vi "verify parameters in range.vi"(8 "error in (no error)":errorcluster, 11 "Simulated_CCD_Camera in":refnum<class "Simulated Camera.lvclass">) -> (0 "error out":errorcluster, 3 "Simulated_CCD_Camera out":refnum<class "Simulated Camera.lvclass">)   [LabVIEW 2018, in "Simulated Camera.lvclass"]
doc: "Verify if the parameters of the camera are in range\n\nThe operating parameters of the CCDs must be within a predefined range. This function verifies if the values provided for these parameters meet this specification. If not, ACS will not allow to start an exposure."
uses:
  Simulated Camera.lvclass
  Simulated Camera.lvclass/Simulated Camera.ctl
panel:
  out "new operation mode":T1
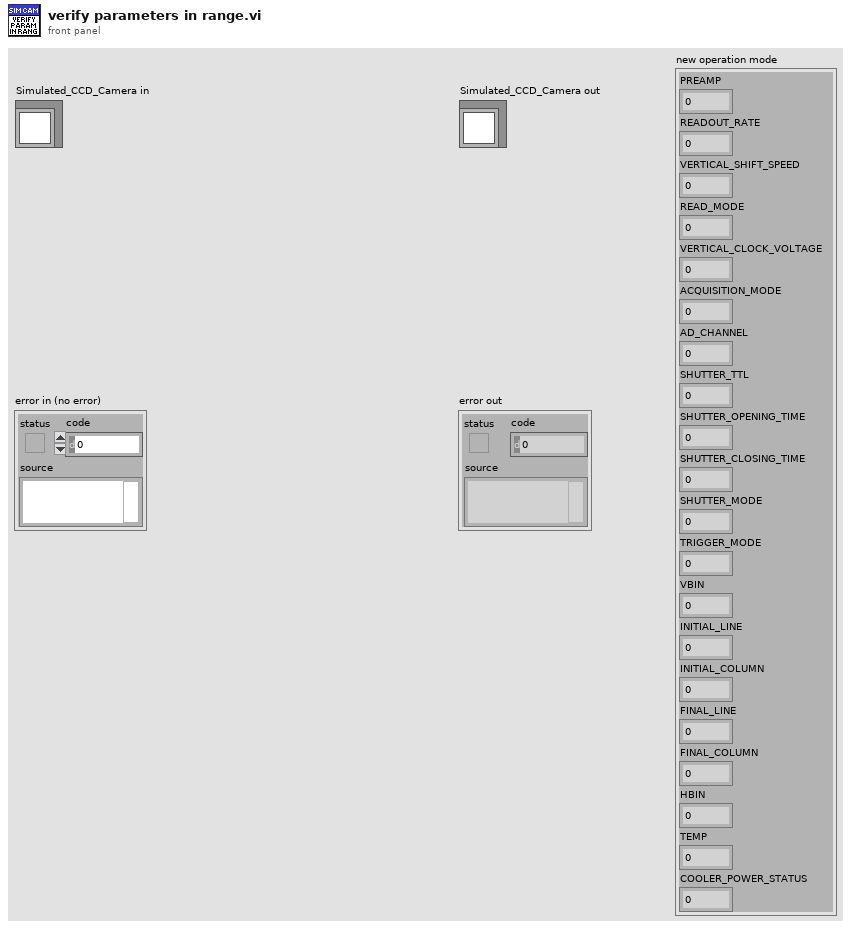
[diagram p1: front panel]
types:
  T1 = cluster{"PREAMP":u16, "READOUT_RATE":u16, "VERTICAL_SHIFT_SPEED":u16, "READ_MODE":u16, "VERTICAL_CLOCK_VOLTAGE":u16, "ACQUISITION_MODE":u16, "AD_CHANNEL":u16, "SHUTTER_TTL":u16, "SHUTTER_OPENING_TIME":u16, "SHUTTER_CLOSING_TIME":u16, "SHUTTER_MODE":u16, "TRIGGER_MODE":u16, "VBIN":u16, "INITIAL_LINE":u16, "INITIAL_COLUMN":u16, "FINAL_LINE":u16, "FINAL_COLUMN":u16, "HBIN":u16, "TEMP":u16, "COOLER_POWER_STATUS":u16}
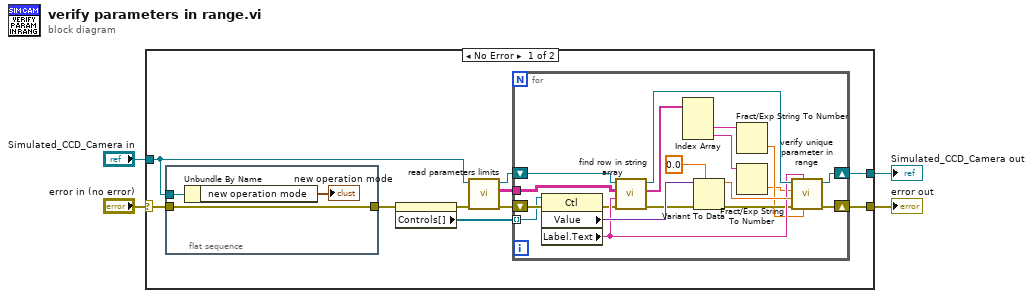
[diagram p0: block diagram]
diagram:
  n1 = case shown="No Error" "error in (no error)" {
    selector: "error in (no error)" -> [w8 w38]
    tunnel: [w14 w38] -> w3
    tunnel: [w13 w37] -> w2
    tunnel: "Simulated_CCD_Camera in" -> [w12 w37]
    frame No Error {
      n2 = flat-sequence {
        tunnel: w12 -> [w17]
        tunnel: w8 -> [w15]
        tunnel: [w15] -> w7
        frame #0 {
          n3 = Unbundle By Name(w17) -> ("new operation mode"=→"new operation mode":T1)
        }
      }
      n4 = property on="new operation mode" class="Clust (strict)"(error in=w7) -> (error out=w6:errorcluster, "Controls[]"=w5:refnum<vi>[])  [unwired: 1 in, 1 out]
      n5 = call "read parameters limits.vi"("error in (no error)"=w6, "Simulated_CCD_Camera in"=w12) -> ("error out"=w11:errorcluster, "limit values spreadsheet"=w10:string[][], "Simulated_CCD_Camera out"=w9:refnum<class "Simulated Camera.lvclass">)  [unwired: 7 in]
      n6 = for {
        shift-right: [w36] -> w14
        shift-left: w11 -> [w21]
        tunnel: w10 -> [w31]
        shift-right: [w32] -> w13
        shift-left: w9 -> [w29]
        tunnel: w5 -> [w18] mode=indexing
        n7 = property class="Ctl"(reference=w18, error in=w21) -> (error out=w23:errorcluster, "Value"=w35:variant, "Label.Text"=w25:string)  [unwired: 1 out]
        n8 = call "find row in string array.vi"("error in (no error)"=w23, "parameter name"=w25, "limit values"=w31, "Simulated_CCD_Camera in"=w29) -> ("error out"=w22:errorcluster, "row"=w30:string[], "Simulated_CCD_Camera out"=w28:refnum<class "Simulated Camera.lvclass">)  [unwired: 5 in]
        n9 = Index Array(array=w30) -> (element #2=w27:string, element #3=w26:string)  [unwired: 3 in, 1 out]
        n10 = Variant To Data(error in=w22, type=0.0, Variant=w35) -> (data=w33:dbl, error out=w24:errorcluster)
        n11 = Fract/Exp String To Number(string=w27) -> (number=w20:dbl)  [unwired: 3 in, 1 out]
        n12 = Fract/Exp String To Number(string=w26) -> (number=w19:dbl)  [unwired: 3 in, 1 out]
        n13 = call "verify unique parameter in range.vi"("lower limit"=w20, "parameter name"=w25, "error in (no error)"=w24, "value"=w33, "upper limit"=w19, "Simulated_CCD_Camera in"=w28) -> ("error out"=w36:errorcluster, "Simulated_CCD_Camera out"=w32:refnum<class "Simulated Camera.lvclass">)  [unwired: 4 in]
      }
    }
    frame Error {
    }
  }
  "error out" <- w3
  "Simulated_CCD_Camera out" <- w2
